vi "test_counter.vi"() -> ()   [LabVIEW 2016]
uses:
  <vilib>/rvi/DesktopExecutionNode/Execution/niFpgaDEN_Execute.vi
  <vilib>/rvi/DesktopExecutionNode/DesktopExecutionNode.xnode
panel:
  in  "version2":bool
  out "pulses":cluster{"maxPulse":bool, "maxReached":bool}[](array[cluster])
  out "indices":cluster{"index":u16, "next":u16}[](array[cluster])
  in  "reset":i32=52
  in  "maxCount":u16=16
  in  "simTime":i32=80
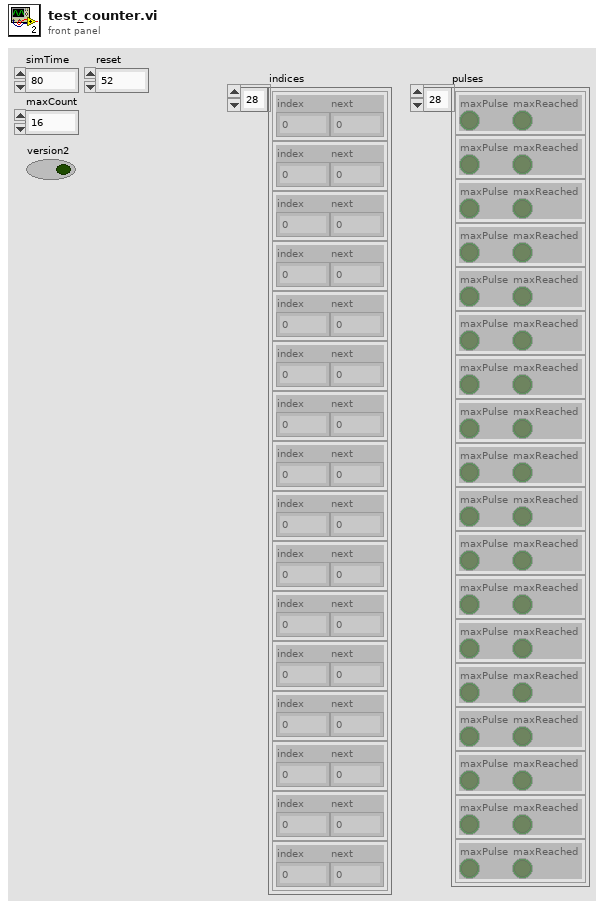
[diagram p1: front panel]
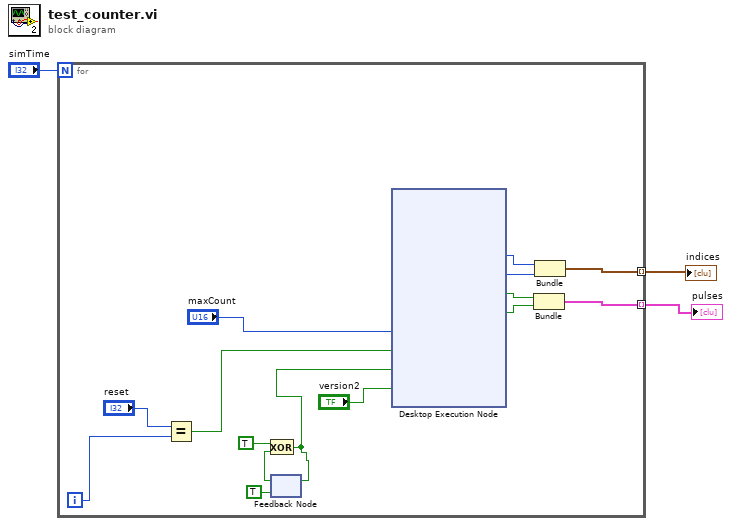
[diagram p0: block diagram]
diagram:
  n1 = for {
    N: "simTime" -> [_]
    tunnel: [w12] -> w2 mode=indexing
    tunnel: [w9] -> w1 mode=indexing
    i -> [w17]
    n2 = Equal?(x="reset", y=w17) -> (x = y?=w16:bool)
    n3 = feedback #1(TRUE) -> (w8:bool)
    n4 = Exclusive Or(1:w8, 2:TRUE ("x")) -> (0:w5:bool)
    n5 = feedback-in #1(w5) -> ()
    n6 = xnode "Desktop Execution Node"("maxCount"="maxCount", "reset"=w16, "doStep"=w5, "version2"="version2") -> ("index"=w14:u16, "next"=w13:u16, "maxPulse"=w11:bool, "maxReached"=w10:bool)  [unwired: 1 in, 1 out]
    n7 = Bundle("maxPulse"=w11, "maxReached"=w10) -> (w9:cluster{"maxPulse":bool, "maxReached":bool})  [unwired: 1 in]
    n8 = Bundle("index"=w14, "next"=w13) -> (w12:cluster{"index":u16, "next":u16})  [unwired: 1 in]
  }
  "indices" <- w2
  "pulses" <- w1
